vi "PZT To Target.vi"(8 "error in (no error)":errorcluster caption="错误输入（无错误）", 10 "Taget":dbl, 11 "VISA resource name":refnum<visa-resource-name> caption="VISA资源名称") -> (0 "错误输出":errorcluster, 3 "VISA资源名称输出":refnum<visa-resource-name>)   [LabVIEW 2014]
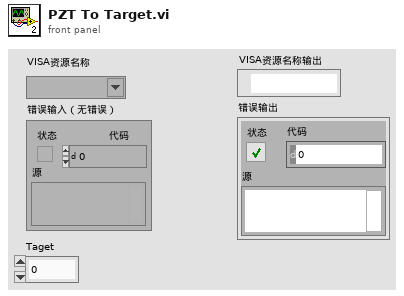
[diagram p1: front panel]
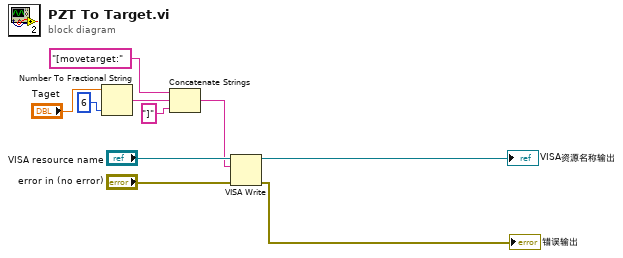
[diagram p0: block diagram]
diagram:
  n1 = Number To Fractional String(number="Taget", precision (6)=i16 6 ("精度(6)")) -> (F-format string=w5:string)  [unwired: 2 in]
  n2 = Concatenate Strings("[movetarget:" ("写入缓冲区"), w5, "]" ("字符串")) -> (w1:string)
  n3 = VISA Write(VISA resource name="VISA resource name", write buffer=w1, error in (no error)="error in (no error)") -> (VISA resource name out=→"VISA资源名称输出":refnum<visa-resource-name>, error out=→"错误输出":errorcluster)  [unwired: 1 out]
